vi "Tosca-Analog Input Monitor Thread.vi"(0 "IPC":T1) -> (15 "error out":errorcluster)   [LabVIEW 2020]
uses:
  IPC VIs/Tosca-IPC.ctl
  Classes/Parameters/Parameters.lvclass
  Digital Input VIs/Tosca-DI Queue Data.ctl
  Digital Input VIs/Tosca-Input Event.ctl
  Digital Input VIs/Tosca-Input Criterion.ctl
  epl-vi-lib/Utility VIs/Type Defs/Logic State.ctl
  Typedefs/Tosca-Accumulator.ctl
  Typedefs/Tosca-State AODO.ctl
  Typedefs/Tosca-AO Runtime.ctl
  Typedefs/Tosca-DO Runtime.ctl
  epl-vi-lib/Signal Synthesis VIs/4th Generation/Classes/SignalManager/SignalManager.lvclass
  Typedefs/Tosca-Synapse Start Data.ctl
  IPC VIs/Tosca-Message.ctl
  IPC VIs/Tosca-Message Action.ctl
  Typedefs/Tosca-Thread Type.ctl
  Imaging VIs/Tosca-2P-Notifier Data.ctl
  Typedefs/Tosca-MATLAB Queue Data.ctl
  Visual Stim VIs/Tosca-Grating.ctl
  Visual Stim VIs/Tosca-Grating Type.ctl
  Typedefs/Tosca-File IO Notification.ctl
  epl-vi-lib/TCP VIs/TCP Params.ctl
  813913c8-8ba4-455b-9e6f-c9f1d86417b5.vi
  epl-vi-lib/TCP VIs/TCP Write.vi
  Sub VIs/Tosca-Globals.vi
  epl-vi-lib/Utility VIs/File IO VIs/Read Write Anything/Read Anything.vi
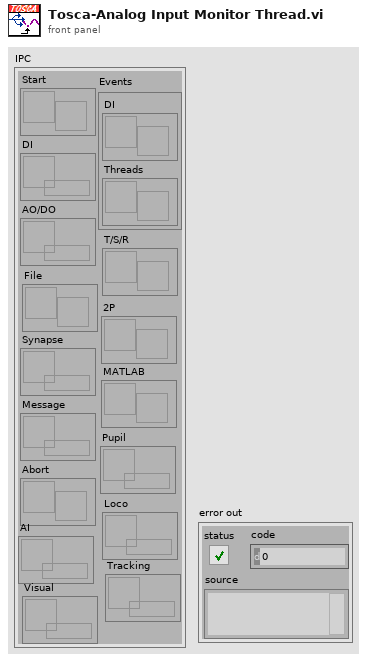
[diagram p1: front panel]
types:
  T1 = typedef "Tosca-IPC.ctl" = cluster{"Start":refnum<notifier>, "DI":refnum<queue>, "AO/DO":refnum<queue>, "Synapse":refnum<queue>, "Message":refnum<queue>, "Abort":refnum<notifier>, "Events":cluster{"DI":refnum<user-event>, "Threads ":refnum<user-event>}, "T/S/R":refnum<notifier>, "2P":refnum<notifier>, "MATLAB":refnum<notifier>, "Pupil":refnum<queue>, "Loco":refnum<queue>, "AI":refnum<queue>, "Tracking":refnum<queue>, "Visual":refnum<queue>, "File":refnum<notifier>}
  T2 = enum16{"big-endian, network order", "native, host order", "little-endian"}
  T3 = typedef "TCP Params.ctl" = cluster{"IP Address":string, "Port":i32}
  T4 = typedef "Tosca-Thread Type.ctl" = enum16{"None", "AODO", "Masker", "ET", "Imaging", "Pupil", "AI", "DI", "Camera", "TTL out", "Loco", "Visual"}
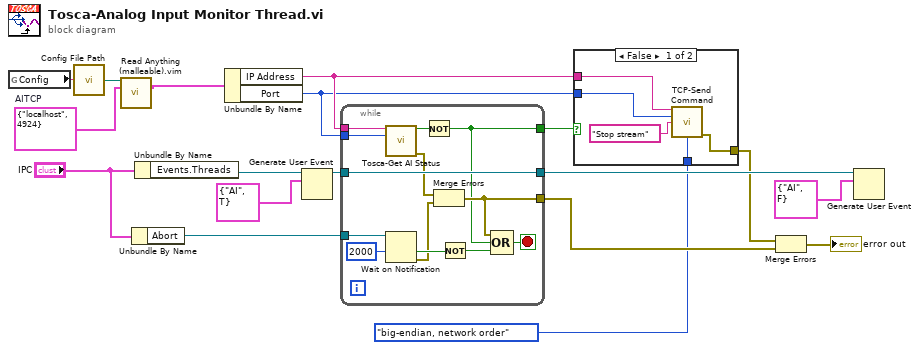
[diagram p0: block diagram]
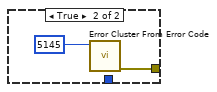
[diagram p2: hidden frame]
diagram:
  w3 = T3 {"IP Address"="localhost", "Port"=4924}  # AITCP
  n1 = global read "Tosca-Globals.vi" "Config"() -> (w5:string)
  n2 = call "Config File Path.vi"("AppName"=w5) -> ("Default config file name"=w4:path)
  n3 = call "Read Anything (malleable).vim"("Config file path"=w4, "Options in"=w3) -> ("Options out"=w2:T3)  [unwired: 10 in, 3 out]
  n4 = Unbundle By Name("IPC") -> ("Abort"=w13:refnum<notifier>)
  n5 = Unbundle By Name("IPC") -> ("Events.Threads"=w18:refnum<user-event>)
  n6 = Unbundle By Name(w2) -> ("IP Address"=w7:string, "Port"=w6:i32)
  n7 = Generate User Event(user event=w18, event data cluster=cluster{"ID":T4, "Running":bool} {"ID"=enum."AI", "Running"=TRUE} ("event data")) -> (user event out=w16:refnum<user-event>)  [unwired: 2 in, 1 out]
  n8 = while {
    tunnel: w16 -> [w31]
    tunnel: [w31] -> w15
    tunnel: w13 -> [w28]
    tunnel: w7 -> [w25]
    tunnel: w6 -> [w24]
    tunnel: [w19] -> w10
    tunnel: [w20] -> w9
    stop <- w26 stop-if-true
    n9 = call "Tosca-Get AI Status.vi"("IP Address"=w25, "Port"=w24) -> ("Recording"=w23:bool, "error out"=w22:errorcluster)  [unwired: 12 in]
    n10 = Wait on Notification(notifier=w28, timeout in ms (-1)=2000) -> (timed out?=w30:bool, error out=w21:errorcluster)  [unwired: 2 in, 2 out]
    n11 = Not(x=w23) -> (.not. x?=w19:bool)
    n12 = Merge Errors(w22, w21) -> (w20:errorcluster)
    n13 = Not(x=w30) -> (.not. x?=w27:bool)
    n14 = Compound Arithmetic op=OR(w20, w19, w27) -> (w26:bool)
  }
  n15 = case shown="False" w10 {
    tunnel: [w33 w37] -> w8
    tunnel: w7 -> [w35 _]
    tunnel: w6 -> [w34 _]
    tunnel: T2."big-endian, network order" ("byte order") -> [w32 _]
    frame False {
      n16 = call "TCP-Send Command.vi"("PXI Address"=w35, "Port"=w34, "Command"="Stop stream", "byte order"=w32) -> ("error out"=w33:errorcluster)  [unwired: 11 in]
    }
    frame True {
      n17 = call <vilib>:"Error Cluster From Error Code.vi"("error code (0)"=5145) -> ("error out"=w37:errorcluster)  [unwired: 8 in]
    }
  }
  n18 = Merge Errors(w8, w9) -> (→"error out":errorcluster)
  n19 = Generate User Event(user event=w15, event data cluster=cluster{"ID":T4, "Running":bool} {"ID"=enum."AI", "Running"=FALSE} ("event data")) -> ()  [unwired: 2 in, 2 out]
